vi "Shift Zero (multiple).vi"(8 "error in (no error)":errorcluster, 10 "Zero x index":dbl, 11 "XY-data":cluster{"X-array":dbl[], "Y-array":dbl[]}[](array[cluster])) -> (0 "error out":errorcluster, 3 "Shifted XY-data out":cluster{"X-array":dbl[], "Y-array":dbl[]}[](array[cluster]) {"Y-array" format="%.2p"; "X-array" format="%.2p"})   [LabVIEW 2019, in "xy_utilities.lvlib"]
doc: "Shift the zero value of the x array by giving a new fractional x index.\n\nWire data to the data input to determine the polymorphic instance to use or manually select the instance."
uses:
  xy_utilities.lvlib
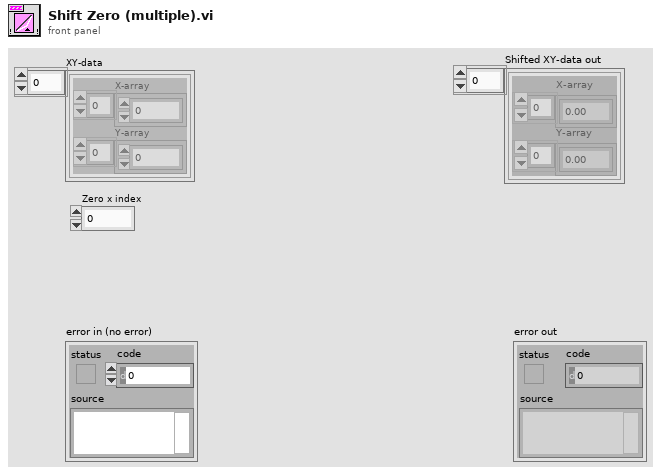
[diagram p1: front panel]
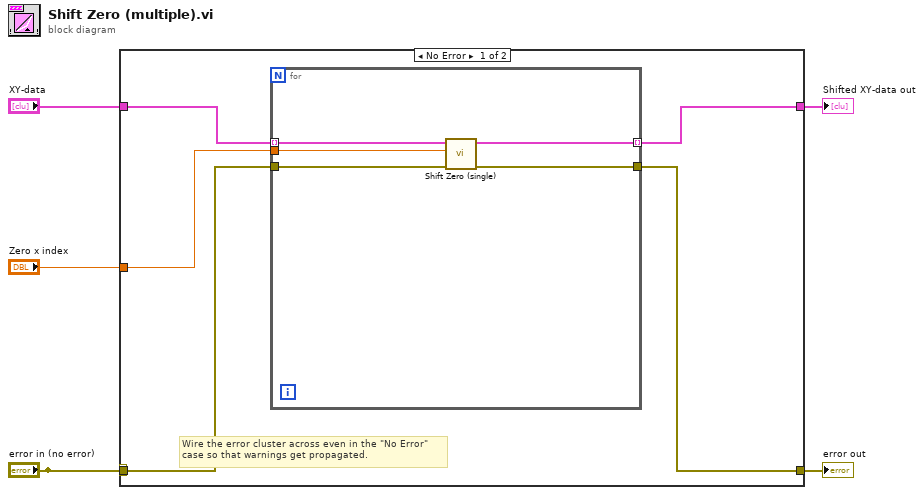
[diagram p0: block diagram]
diagram:
  n1 = case shown="No Error" "error in (no error)" {
    selector: "error in (no error)" -> [_ w17]
    tunnel: [w6 w17] -> w5
    tunnel: "XY-data" -> [w8 w16]
    tunnel: [w7 w16] -> w1
    tunnel: "Zero x index" -> [w9 _]
    tunnel: "error in (no error)" -> [w10 _]
    frame No Error {
      # "Wire the error cluster across even in the \"No Error\"\ncase so that warnings get propagated."
      n2 = for {
        tunnel: w10 -> [w15]
        tunnel: w9 -> [w14]
        tunnel: w8 -> [w13] mode=indexing
        tunnel: [w12] -> w7 mode=indexing
        tunnel: [w11] -> w6
        n3 = call "Shift Zero (single).vi"("error in (no error)"=w15, "Zero x index"=w14, "XY-data"=w13) -> ("error out"=w11:errorcluster, "Shifted XY-data out"=w12:cluster{"X-array":dbl[], "Y-array":dbl[]})  [unwired: 7 in]
      }
    }
    frame Error {
    }
  }
  "error out" <- w5
  "Shifted XY-data out" <- w1
